vi "Global_seed.vi"() -> ()   [LabVIEW 2014]
panel:
  out "seed_v_out":dbl[](array[numeric])
  out "seed_h_out":dbl[](array[numeric])
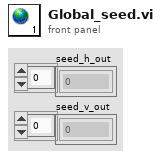
[diagram p1: front panel]
diagram:
